vi "save_txpower.vi"(0 "Apeak":dbl[](array[numeric]), 1 "Apeakpos":dbl[](array[numeric]), 2 "Apeaknext":dbl[](array[numeric]), 3 "Anextpos":dbl[](array[numeric]), 4 "Bpeak":dbl[](array[numeric]), 5 "Bpeakpos":dbl[](array[numeric]), 6 "PATH":string, 7 "Bpeaknext":dbl[](array[numeric]), 8 "Tabsize":dbl, 9 "Bnextpos":dbl[](array[numeric]), 10 "FreqTab":dbl[](array[numeric]), 11 "RApeak":dbl[](array[numeric]), 13 "RApos":dbl[](array[numeric]), 18 "RBpos":dbl[](array[numeric]), 19 "RBpeak":dbl[](array[numeric])) -> ()   [LabVIEW 2015]
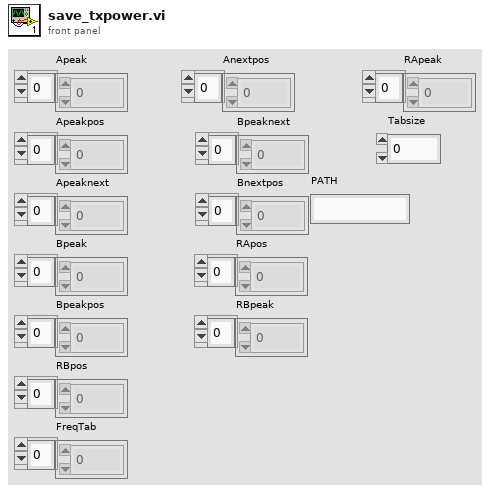
[diagram p1: front panel]
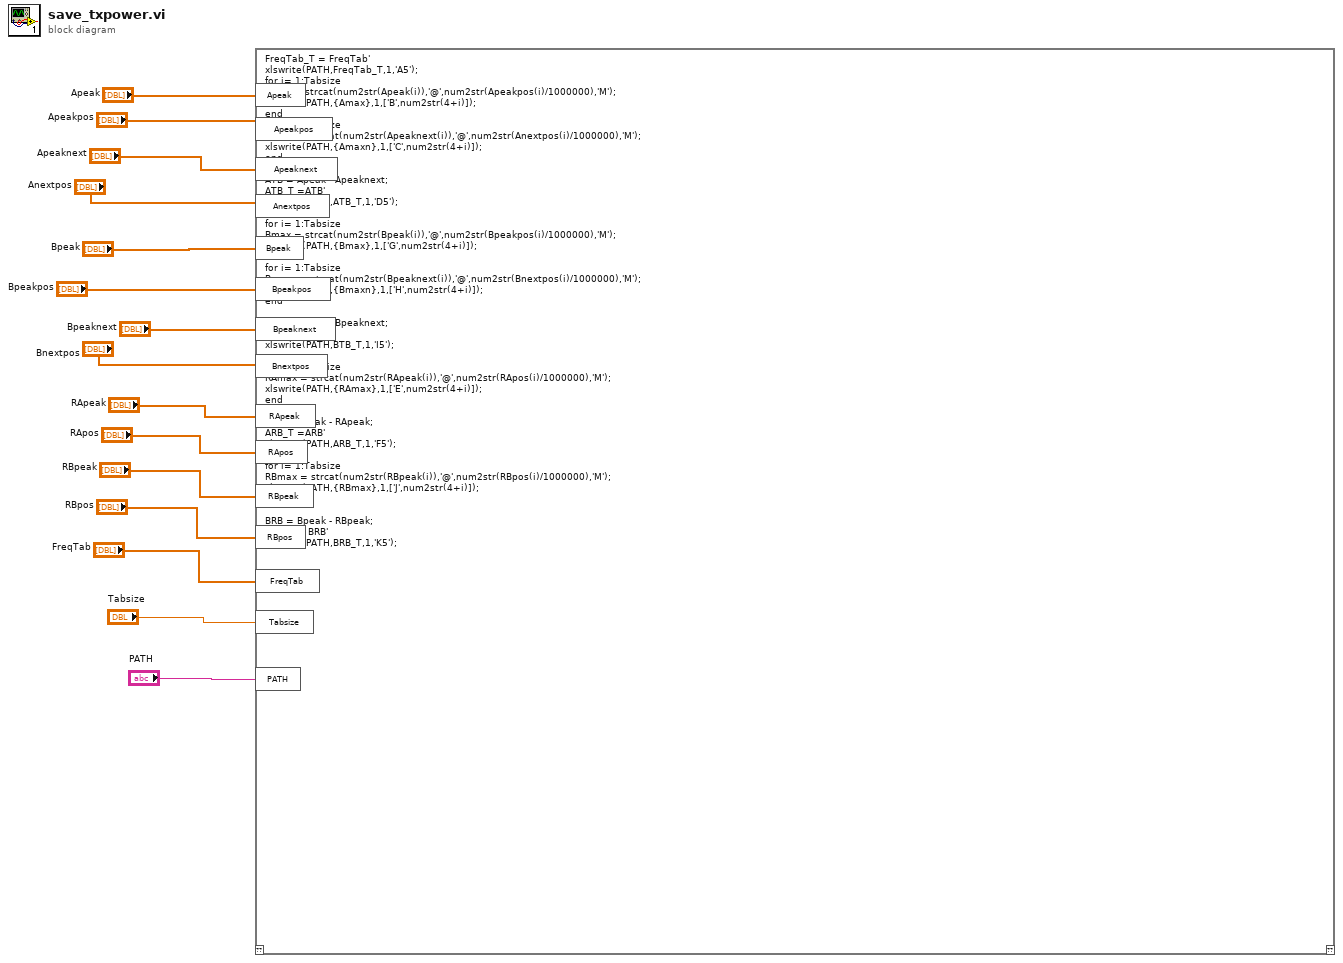
[diagram p0: block diagram]
diagram:
  n1 = script code="FreqTab_T = FreqTab'\nxlswrite(PATH,FreqTab_T,1,'A5');\nfor i= 1:Tabsize\nAmax = strcat(num2str(Apeak(i)),'@',num2str(Apeakpos(i)/1000000),'M');\nxlswrite(PATH,{Amax},1,['B',num2str(4+i)]);\nend\nfor i= 1:Tabsize\nAmaxn = strcat(num2str(Apeaknext(i)),'@',num2str(Anextpos(i)/1000000),'M');\nxlswrite(PATH,{Amaxn},1,['C',num2str(4+i)]);\nend\n\nATB = Apeak - Apeaknext;\nATB_T =ATB'\nxlswrite(PATH,ATB_T,1,'D5');\n\nfor i= 1:Tabsize\nBmax = strcat(num2str(Bpeak(i)),'@',num2str(Bpeakpos(i)/1000000),'M');\nxlswrite(PATH,{Bmax},1,['G',num2str(4+i)]);\nend\nfor i= 1:Tabsize\nBmaxn = strcat(num2str(Bpeaknext(i)),'@',num2str(Bnextpos(i)/1000000),'M');\nxlswrite(PATH,{Bmaxn},1,['H',num2str(4+i)]);\nend\n\nBTB = Bpeak - Bpeaknext;\nBTB_T =BTB'\nxlswrite(PATH,BTB_T,1,'I5');\n\nfor i= 1:Tabsize\nRAmax = strcat(num2str(RApeak(i)),'@',num2str(RApos(i)/1000000),'M');\nxlswrite(PATH,{RAmax},1,['E',num2str(4+i)]);\nend\n\nARB = Apeak - RApeak;\nARB_T =ARB'\nxlswrite(PATH,ARB_T,1,'F5');\n\nfor i= 1:Tabsize\nRBmax = strcat(num2str(RBpeak(i)),'@',num2str(RBpos(i)/1000000),'M');\nxlswrite(PATH,{RBmax},1,['J',num2str(4+i)]);\nend\n\nBRB = Bpeak - RBpeak;\nBRB_T = BRB'\nxlswrite(PATH,BRB_T,1,'K5');"("Apeak"="Apeak", "Apeakpos"="Apeakpos", "Apeaknext"="Apeaknext", "Anextpos"="Anextpos", "Bpeak"="Bpeak", "Bpeakpos"="Bpeakpos", "Bpeaknext"="Bpeaknext", "Bnextpos"="Bnextpos", "RApeak"="RApeak", "RApos"="RApos", "RBpeak"="RBpeak", "RBpos"="RBpos", "FreqTab"="FreqTab", "Tabsize"="Tabsize", "PATH"="PATH") -> ()  [unwired: 1 in, 1 out]
